vi "Live Capture Functional Stack.6.64bit.vi"() -> ()   [LabVIEW 2014]
uses:
  subvis/Stack Track.ctl
  subvis/Stack_State.ctl
  Desktop/camtiff/ctiff.llb/__CTIFFNewFileAndStyleUINT16.vi
  Desktop/camtiff/ctiff.llb/__CTIFFAddNewPageUINT16.vi
  CameraControlTypeDef.ctl
panel:
  in  "Slit Width / Lines 2":sgl=150.0
  out "Frame Index":i32
  in  "Internal Line Interval":dbl
  in  "Readout Direction":sgl(ring)=1.0 items=["Forward"=1, "Backward"=2]
  in  "Trigger Mode":sgl(ring)=1.0 items=["Normal"=1, "Start "=6]
  in  "Trigger Source":sgl(ring)=2.0 items=["Internal"=1, "External"=2]
  out "State":T1=enum."Start Sequence"
  out "Image":u16[][](graph)
  out "Saving":bool
  in  "AutoIncrement":bool=TRUE
  in  "Path":path=path "C:/Users/spim/Desktop/Craig Cap/temp/a.tiff"
  out "error out":errorcluster
  in  "stop":bool
  out "Total Frames":i32
  out "Elapsed Time":u32
  out "Software FPS":dbl
  out "Camera FPS":dbl
  in  "H Offset":i32 min=0 max=0
  in  "H Width":i32 min=0 max=0
  out "SMD":dbl
  out "SHO":i32
  in  "V Offset":i32 min=0 max=0
  in  "V Width":i32 min=0 max=0
  in  "Binning":u16(ring) items=["1x1"=1, "2x2"=2, "4x4"=4]
  out "SHW":i32
  out "SVO":i32
  out "SVW":i32
  in  "Scan Mode":dbl min=0.0 max=0.0
  in  "Exposure":dbl min=0.0 max=0.0
  out "EXP":dbl
  out "Camera Model":string
  out "Camera Version":string
  out "Camera Serial":string
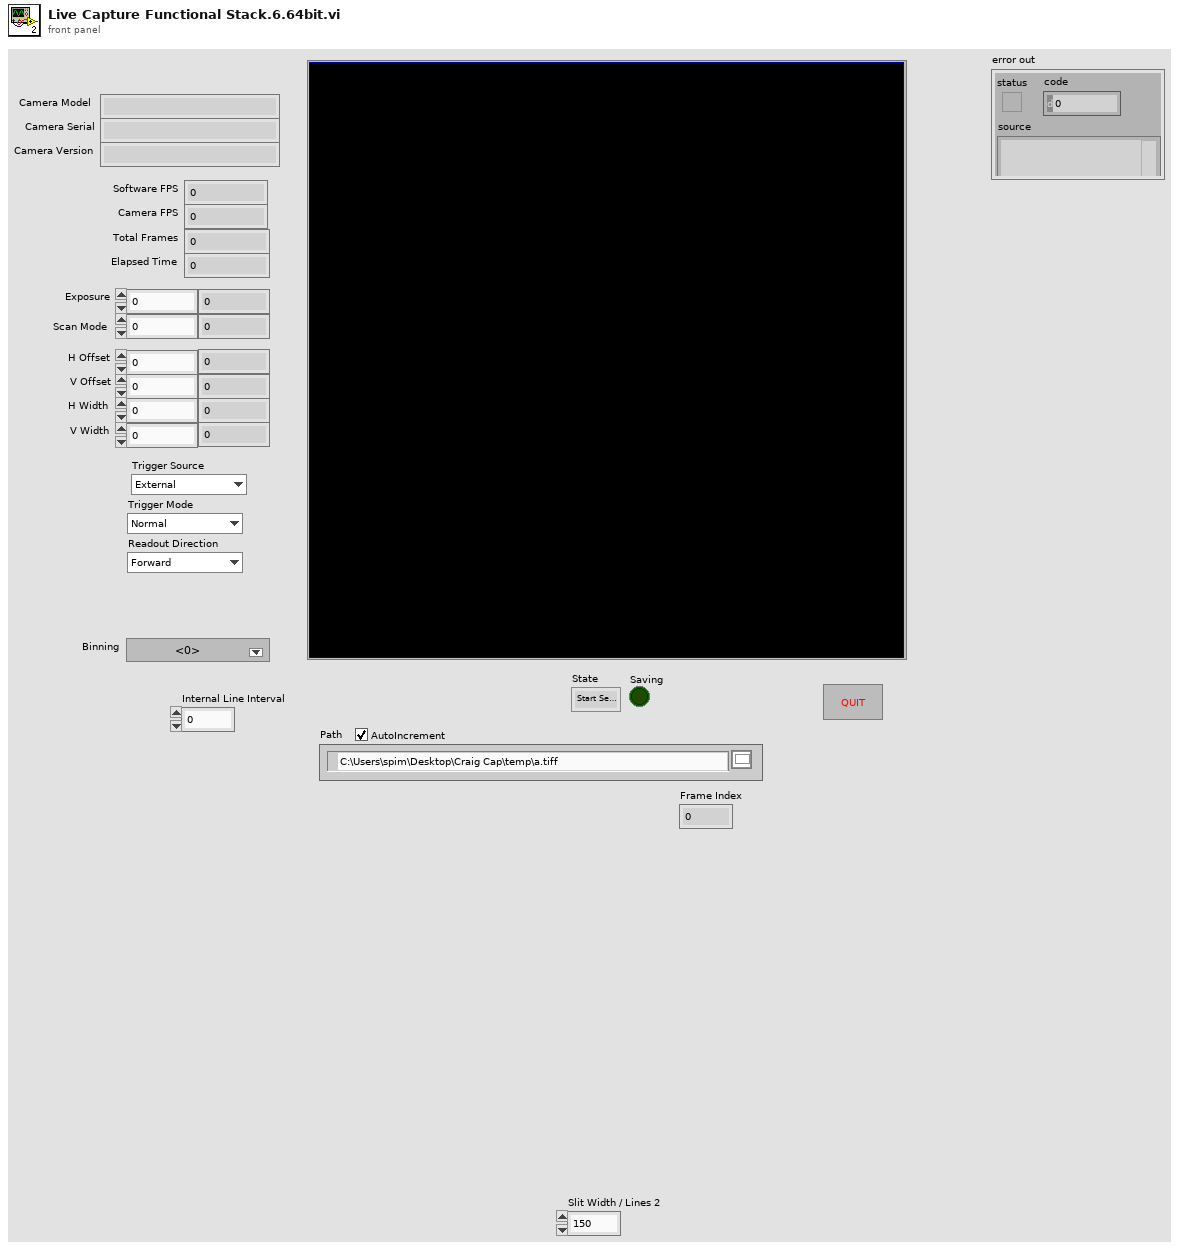
[diagram p1: front panel]
types:
  T1 = typedef "Stack Track.ctl" = enum16{"Idle", "Start Sequence", "Read Disk", "STOP", "Collecting", "End"}
  T2 = typedef "CameraControlTypeDef.ctl" = enum16{"Ram Record", "HardDisk Record", "Disengage Update", "Update", "Idle"}
  T3 = typedef "Stack_State.ctl" = cluster{"State":T1, "Stack Number":i32, "Image":u16[][]}
  T4 = cluster{"Model":string, "Camera ID":string, "Firmware":string}
  T5 = cluster{"Value":i32, "Minimum":i32, "Maximum":i32, "Increment":i32}
  T6 = cluster{"height":u32, "width":u32, "datatype":u32}
  T7 = cluster{"H Offset":i32, "V Offset":i32, "H Width":i32, "V Width":i32}
  T8 = enum8{"Enabled", "Disabled", "Disabled and Grayed Out"}
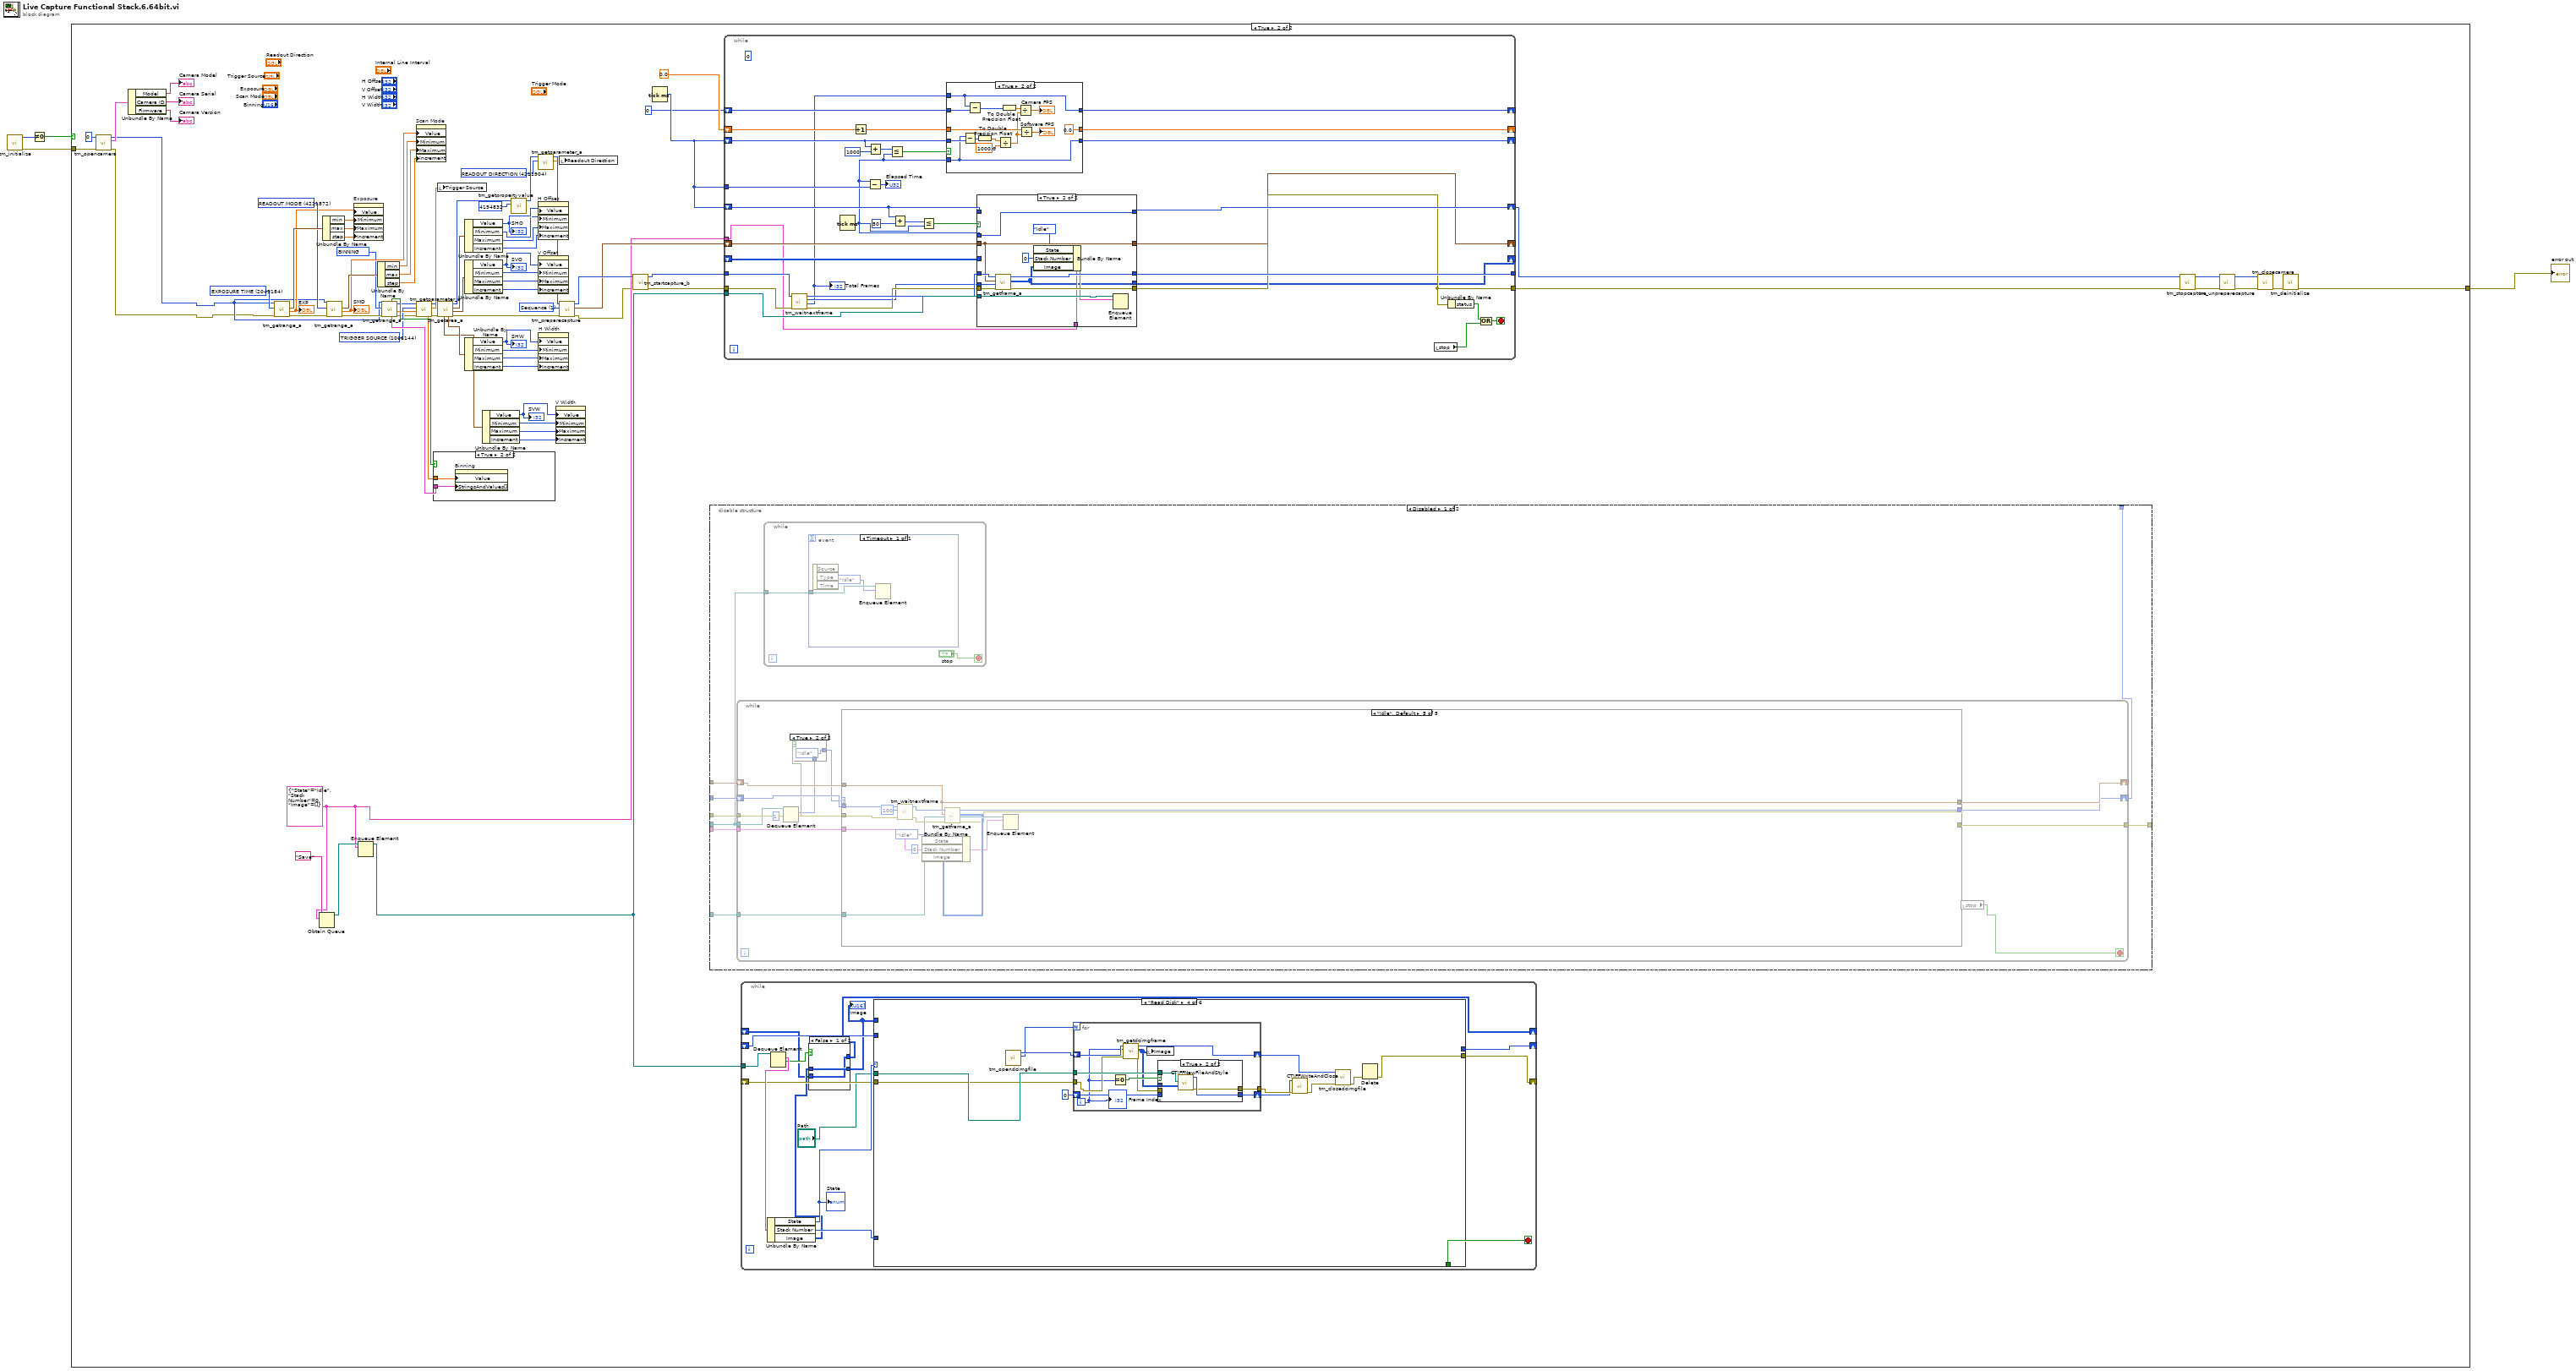
[diagram p0: block diagram]
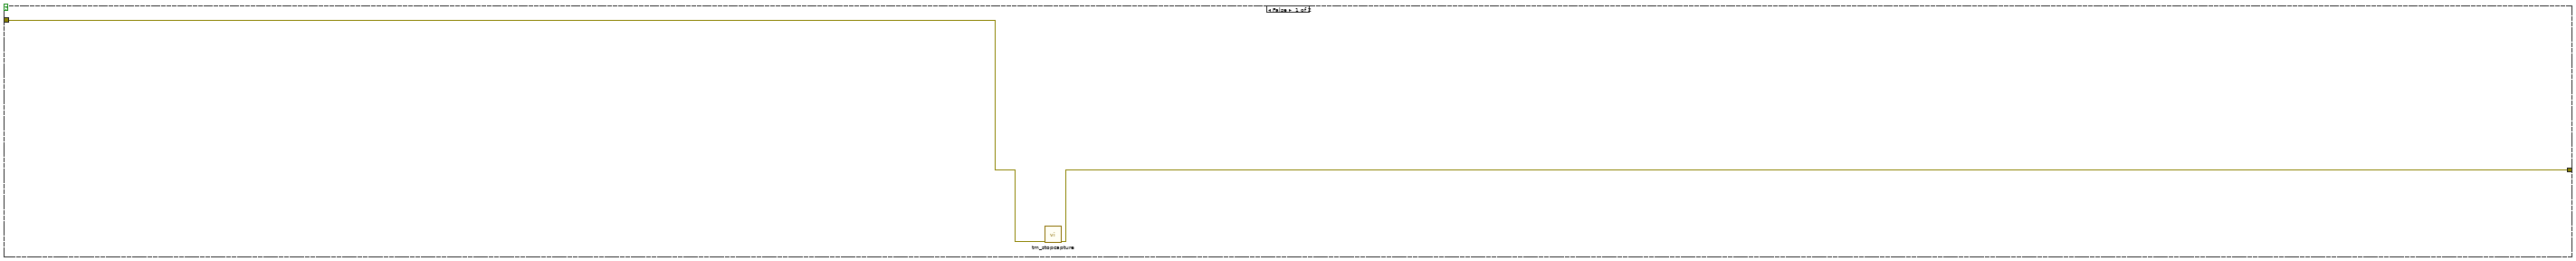
[diagram p2: hidden frame]
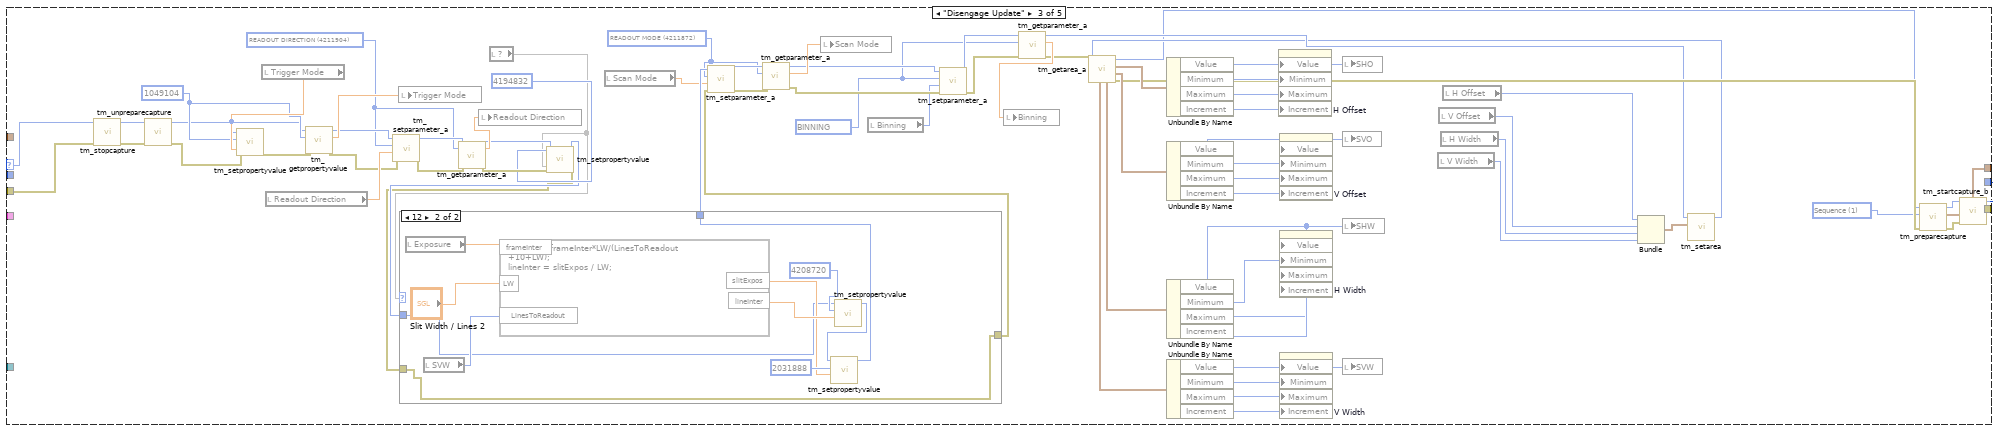
[diagram p8: hidden frame]
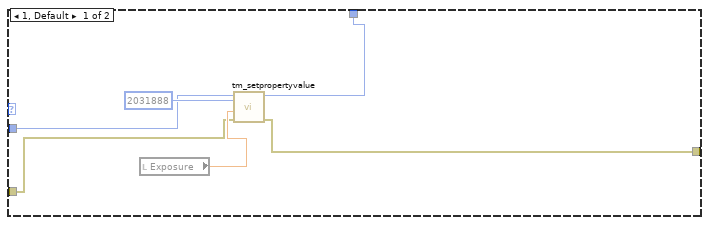
[diagram p9: hidden frame]
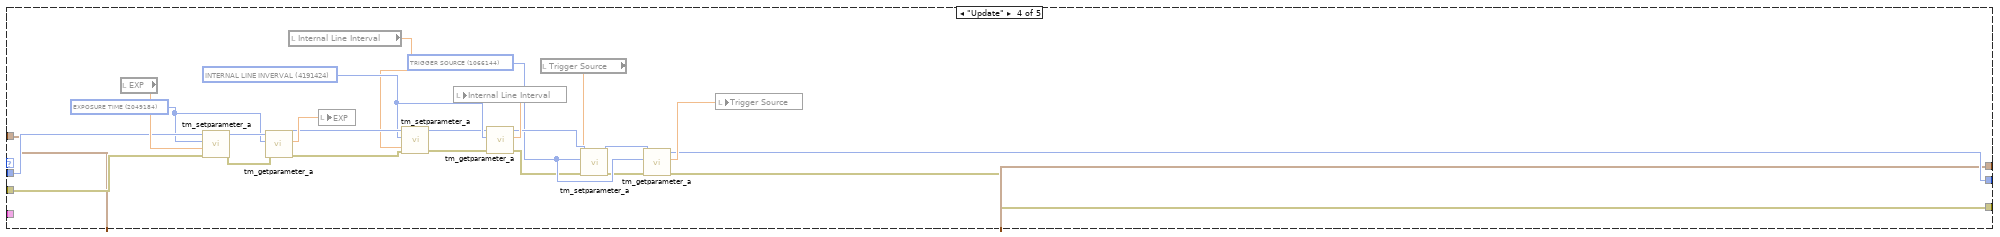
[diagram p10: hidden frame]
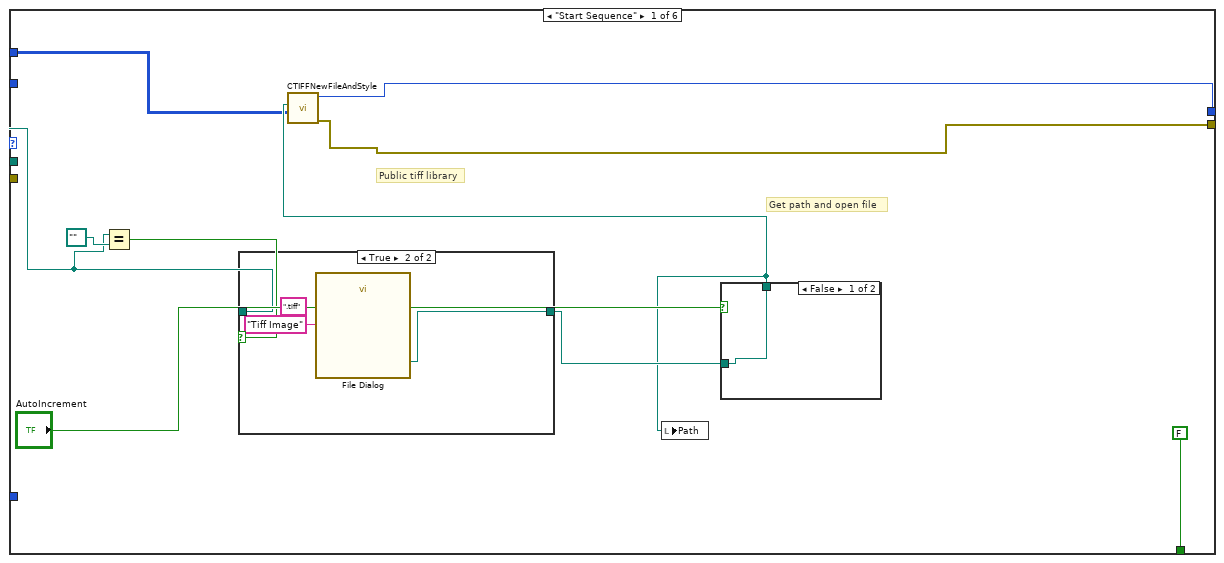
[diagram p13: hidden frame]
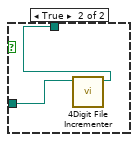
[diagram p15: hidden frame]
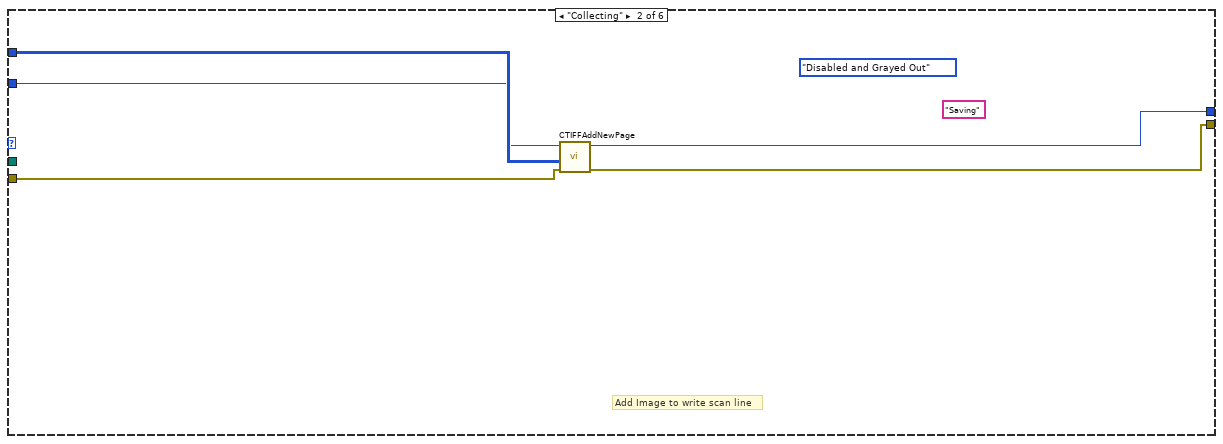
[diagram p16: hidden frame]
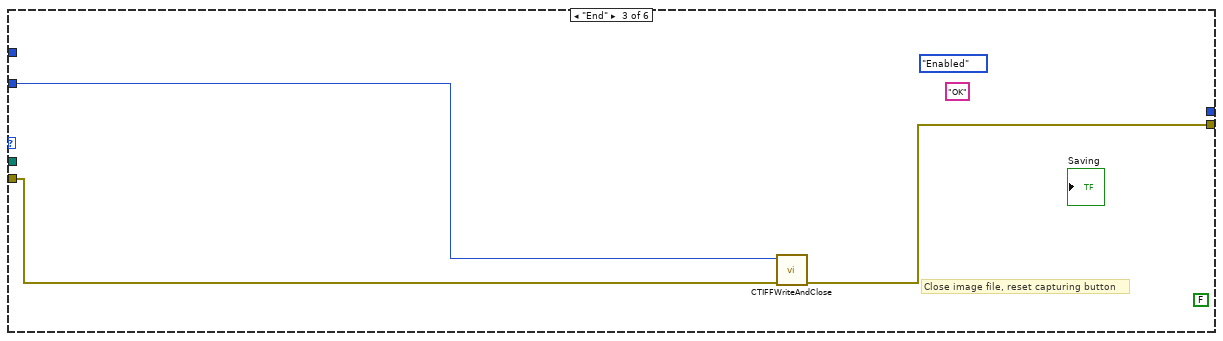
[diagram p17: hidden frame]
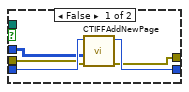
[diagram p18: hidden frame]
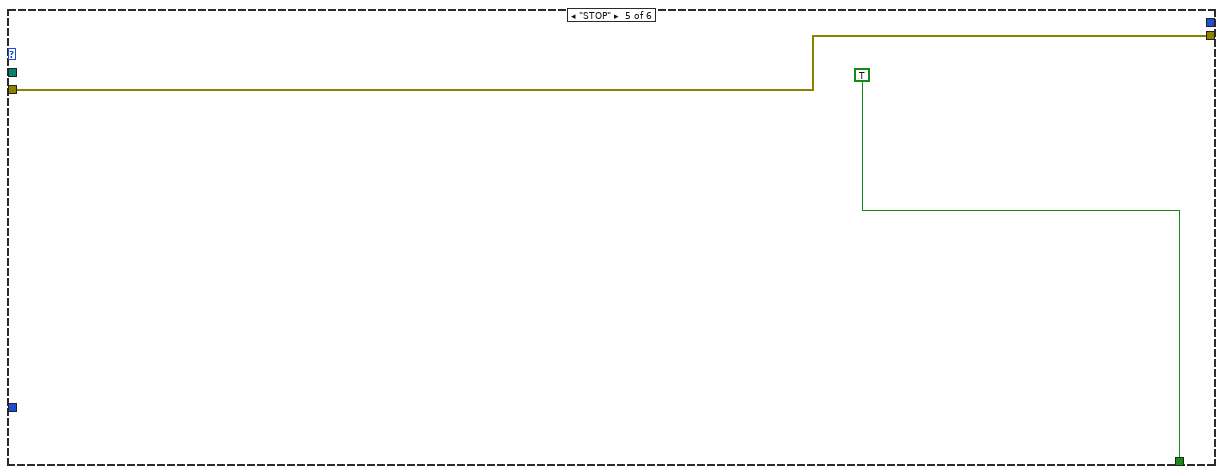
[diagram p19: hidden frame]
diagram:
  n1 = call <userlib>:"tm_initialize.vi"() -> ("error out"=w2:errorcluster, "Number Of Cameras"=w1:u32)  [unwired: 8 in, 2 out]
  n2 = Not Equal To 0?(x=w1) -> (x != 0?=w4:bool)
  n3 = case shown="True" w4 {
    tunnel: [w5 w83] -> w3
    tunnel: w2 -> [w6 w86]
    frame False {
      n4 = call <userlib>:"tm_stopcapture.vi"("error in (no error)"=w6) -> ("error out"=w5:errorcluster)  [unwired: 9 in, 1 out]
    }
    frame True {
      w19 = u32 4211904 items=["SENSOR MODE"=4212128, "CCD MODE"=4212384, "READOUT MODE"=4211872, "ACTIVE VIEW INDEX"=4343136, "BITS PER CHANNEL"=4342976, "IMAGE PIXEL TYPE"=4343296, "BINNING"=4215968, "EXPOSURE TIME"=2049184, "CONTRAST GAIN"=3163312, "CONTRAST OFFSET"=3163328, "LIGHT MODE"=2114720, "SENSITIVITY"=2114992, "PHOTON IMAGING MODE"=2115200, "HIGH DYNAMIC RANGE MODE"=3163360, "WHITE BALANCE"=3163568, "TEMPERATURE"=2115232, "TEMPERATURE TARGET"=2115264, "SENSOR COOLER FAN"=2115296, "LINEBUNDLE HEIGHT"=4212192, "MECHANICAL SHUTTER"=2115488, "BACK FOCUS POSITION"=8422304, "TRIGGER CONNECTOR"=1066432, "TRIGGER SOURCE"=1066144, "OUTPUT TRIGGER SOURCE"=1852576, "TRIGGER GLOBAL EXPOSURE"=2049680, "FIRST TRIGGER BEHAVIOR"=2049696, "CHANNEL SYNC"=1852352, "READOUT DIRECTION"=4211904, "PRE HSYNC COUNT"=1852704] ("Parameter")
      w28 = u32 1066144 items=["SENSOR MODE"=4212128, "CCD MODE"=4212384, "READOUT MODE"=4211872, "ACTIVE VIEW INDEX"=4343136, "BITS PER CHANNEL"=4342976, "IMAGE PIXEL TYPE"=4343296, "BINNING"=4215968, "EXPOSURE TIME"=2049184, "CONTRAST GAIN"=3163312, "CONTRAST OFFSET"=3163328, "LIGHT MODE"=2114720, "SENSITIVITY"=2114992, "PHOTON IMAGING MODE"=2115200, "HIGH DYNAMIC RANGE MODE"=3163360, "WHITE BALANCE"=3163568, "TEMPERATURE"=2115232, "TEMPERATURE TARGET"=2115264, "SENSOR COOLER FAN"=2115296, "LINEBUNDLE HEIGHT"=4212192, "MECHANICAL SHUTTER"=2115488, "BACK FOCUS POSITION"=8422304, "TRIGGER CONNECTOR"=1066432, "TRIGGER SOURCE"=1066144, "OUTPUT TRIGGER SOURCE"=1852576, "TRIGGER GLOBAL EXPOSURE"=2049680, "FIRST TRIGGER BEHAVIOR"=2049696, "CHANNEL SYNC"=1852352, "READOUT DIRECTION"=4211904, "PRE HSYNC COUNT"=1852704] ("Parameter")
      w12 = T3 {"State"=enum."Idle", "Stack Number"=0, "Image"=[]} ("input cluster")
      w33 = u32 2049184 items=["BINNING"=4215968, "BITS PER CHANNEL"=4342976, "ACTIVE VIEW INDEX"=4343136, "CCD MODE"=4212384, "SENSOR MODE"=4212128, "READOUT MODE"=4211872, "EXPOSURE TIME"=2049184, "CONTRAST GAIN"=3163312, "CONTRAST OFFSET"=3163328, "LIGHT MODE"=2114720, "SENSITIVITY"=2114992, "WHITE BALANCE"=3163568, "PHOTON IMAGING MODE"=2115200, "HIGH DYNAMIC RANGE MODE"=3163360, "TRIGGER SOURCE"=1066144, "TRIGGER ACTIVE"=1066160, "TRIGGER MODE"=1066400, "TRIGGER POLARITY"=1066416, "TRIGGER GLOBAL EXPOSURE"=2049680, "FIRST TRIGGER BEHAVIOR"=2049696, "TRIGGER TIMES"=1066448, "OUTPUT TRIGGER POLARITY"=1852592, "OUTPUT TRIGGER DELAY"=1852624, "OUTPUT TRIGGER PERIOD"=1852640, "TEMPERATURE"=2115232, "TEMPERATURE TARGET"=2115264, "SENSOR COOLER FAN"=2115296, "MECHANICAL SHUTTER"=2115488, "BACK FOCUS POSITION"=8422304, "FRAMEBUNDLE MODE"=4346784, "FRAMEBUNDLE NUMBER"=4346800, "LINEBUNDLE HEIGHT"=4212192, "TRIGGER CONNECTOR"=1066432, "IMAGE PIXEL TYPE"=4343296, "OUTPUT TRIGGER KIND"=1852656, "READOUT DIRECTION"=4211904, "CHANNEL SYNC"=1852352] ("Parameter")
      w34 = u32 4211872 items=["BINNING"=4215968, "BITS PER CHANNEL"=4342976, "ACTIVE VIEW INDEX"=4343136, "CCD MODE"=4212384, "SENSOR MODE"=4212128, "READOUT MODE"=4211872, "EXPOSURE TIME"=2049184, "CONTRAST GAIN"=3163312, "CONTRAST OFFSET"=3163328, "LIGHT MODE"=2114720, "SENSITIVITY"=2114992, "WHITE BALANCE"=3163568, "PHOTON IMAGING MODE"=2115200, "HIGH DYNAMIC RANGE MODE"=3163360, "TRIGGER SOURCE"=1066144, "TRIGGER ACTIVE"=1066160, "TRIGGER MODE"=1066400, "TRIGGER POLARITY"=1066416, "TRIGGER GLOBAL EXPOSURE"=2049680, "FIRST TRIGGER BEHAVIOR"=2049696, "TRIGGER TIMES"=1066448, "OUTPUT TRIGGER POLARITY"=1852592, "OUTPUT TRIGGER DELAY"=1852624, "OUTPUT TRIGGER PERIOD"=1852640, "TEMPERATURE"=2115232, "TEMPERATURE TARGET"=2115264, "SENSOR COOLER FAN"=2115296, "MECHANICAL SHUTTER"=2115488, "BACK FOCUS POSITION"=8422304, "FRAMEBUNDLE MODE"=4346784, "FRAMEBUNDLE NUMBER"=4346800, "LINEBUNDLE HEIGHT"=4212192, "TRIGGER CONNECTOR"=1066432, "IMAGE PIXEL TYPE"=4343296, "OUTPUT TRIGGER KIND"=1852656, "READOUT DIRECTION"=4211904, "CHANNEL SYNC"=1852352] ("Parameter")
      w35 = u32 4215968 items=["BINNING"=4215968, "BITS PER CHANNEL"=4342976, "ACTIVE VIEW INDEX"=4343136, "CCD MODE"=4212384, "SENSOR MODE"=4212128, "READOUT MODE"=4211872, "EXPOSURE TIME"=2049184, "CONTRAST GAIN"=3163312, "CONTRAST OFFSET"=3163328, "LIGHT MODE"=2114720, "SENSITIVITY"=2114992, "WHITE BALANCE"=3163568, "PHOTON IMAGING MODE"=2115200, "HIGH DYNAMIC RANGE MODE"=3163360, "TRIGGER SOURCE"=1066144, "TRIGGER ACTIVE"=1066160, "TRIGGER MODE"=1066400, "TRIGGER POLARITY"=1066416, "TRIGGER GLOBAL EXPOSURE"=2049680, "FIRST TRIGGER BEHAVIOR"=2049696, "TRIGGER TIMES"=1066448, "OUTPUT TRIGGER POLARITY"=1852592, "OUTPUT TRIGGER DELAY"=1852624, "OUTPUT TRIGGER PERIOD"=1852640, "TEMPERATURE"=2115232, "TEMPERATURE TARGET"=2115264, "SENSOR COOLER FAN"=2115296, "MECHANICAL SHUTTER"=2115488, "BACK FOCUS POSITION"=8422304, "FRAMEBUNDLE MODE"=4346784, "FRAMEBUNDLE NUMBER"=4346800, "LINEBUNDLE HEIGHT"=4212192, "TRIGGER CONNECTOR"=1066432, "IMAGE PIXEL TYPE"=4343296, "OUTPUT TRIGGER KIND"=1852656, "READOUT DIRECTION"=4211904, "CHANNEL SYNC"=1852352] ("Parameter")
      w81 = 1 items=["Snap", "Sequence"] ("Capture mode")
      n5 = call <userlib>:"tm_opencamera.vi"("error in (no error)"=w86, "Camera Index"=u32 0) -> ("error out"=w7:errorcluster, "Camera Details"=w47:T4, "Handle out"=w8:u32)  [unwired: 7 in]
      n6 = Unbundle By Name(w47) -> ("Model"=→"Camera Model":string, "Camera ID"=→"Camera Serial":string, "Firmware"=→"Camera Version":string)
      n7 = call <userlib>:"tm_getrange_a.vi"("error in (no error)"=w7, "Parameter"=w33, "Handle in"=w8) -> ("error out"=w42:errorcluster, "default"=w31:dbl, "Range"=w43:cluster{"min":dbl, "max":dbl, "step":dbl})  [unwired: 2 in, 4 out]
      "EXP" <- w31
      n8 = Obtain Queue(name (unnamed)="Save", element data type=w12) -> (queue out=w16:refnum<queue>)  [unwired: 3 in, 2 out]
      n9 = Unbundle By Name(w43) -> ("min"=w78:dbl, "max"=w77:dbl, "step"=w76:dbl)
      n10 = call <userlib>:"tm_getrange_a.vi"("error in (no error)"=w42, "Parameter"=w34, "Handle in"=w8) -> ("error out"=w39:errorcluster, "default"=w40:dbl, "Range"=w41:cluster{"min":dbl, "max":dbl, "step":dbl})  [unwired: 2 in, 4 out]
      "SMD" <- w40
      n11 = property on="Exposure" class="DigNum (strict)"("Value"=w31, "Minimum"=w78, "Maximum"=w77, "Increment"=w76) -> ()  [unwired: 2 in, 2 out]
      n12 = Enqueue Element(queue=w16, element=w12) -> (queue out=w15:refnum<queue>)  [unwired: 2 in, 2 out]
      n13 = Unbundle By Name(w41) -> ("min"=w75:dbl, "max"=w74:dbl, "step"=w73:dbl)
      n14 = call <userlib>:"tm_getrange_a.vi"("error in (no error)"=w39, "Parameter"=w35, "Handle in"=w8) -> ("error out"=w25:errorcluster, "default"=w37:dbl, "Handle out"=w27:u32, "Value Names"=w36:cluster{"Name":string, "Value":dbl}[], "Writable"=w38:bool)  [unwired: 2 in, 2 out]
      n15 = property on="Scan Mode" class="DigNum (strict)"("Value"=w40, "Minimum"=w75, "Maximum"=w74, "Increment"=w73) -> ()  [unwired: 2 in, 2 out]
      n16 = call <userlib>:"tm_getparameter_a.vi"("error in (no error)"=w25, "Parameter"=w28, "Handle in"=w27) -> ("error out"=w24:errorcluster, "Value out"=w29:dbl, "Handle out"=w26:u32)  [unwired: 6 in]
      n17 = case shown="True" w38 {
        tunnel: w36 -> [_ w398]
        tunnel: w37 -> [_ w397]
        frame False {
        }
        frame True {
          n18 = property on="Binning" class="Ring (strict)"("Value"=w397, "StringsAndValues[]"=w398) -> ()  [unwired: 2 in, 2 out]
        }
      }
      n19 = local write "Trigger Source"(w29) -> ()
      n20 = call <userlib>:"tm_getarea_a.vi"("error in (no error)"=w24, "Handle in"=w26) -> ("error out"=w30:errorcluster, "V Offset"=w72:T5, "H Offset"=w53:T5, "Handle out"=w22:u32, "H Width"=w71:T5, "V Width"=w70:T5)  [unwired: 4 in]
      n21 = Unbundle By Name(w53) -> ("Value"=w52:i32, "Minimum"=w51:i32, "Maximum"=w50:i32, "Increment"=w49:i32)
      "SHO" <- w52
      n22 = Unbundle By Name(w72) -> ("Value"=w60:i32, "Minimum"=w69:i32, "Maximum"=w68:i32, "Increment"=w67:i32)
      "SVO" <- w60
      n23 = Unbundle By Name(w71) -> ("Value"=w59:i32, "Minimum"=w66:i32, "Maximum"=w65:i32, "Increment"=w64:i32)
      "SHW" <- w59
      n24 = Unbundle By Name(w70) -> ("Value"=w58:i32, "Minimum"=w63:i32, "Maximum"=w62:i32, "Increment"=w61:i32)
      "SVW" <- w58
      n25 = call <userlib>:"tm_getpropertyvalue.vi"("Property ID"=u32 4194832, "Handle in"=w22) -> ("Handle out"=w21:u32)  [unwired: 7 in, 2 out]
      n26 = call <userlib>:"tm_getparameter_a.vi"("Parameter"=w19, "Handle in"=w21) -> ("Value out"=w18:dbl, "Handle out"=w20:u32)  [unwired: 7 in, 1 out]
      n27 = property on="H Offset" class="DigNum (strict)"("Value"=w52, "Minimum"=w51, "Maximum"=w50, "Increment"=w49) -> ()  [unwired: 2 in, 2 out]
      n28 = property on="V Offset" class="DigNum (strict)"("Value"=w60, "Minimum"=w69, "Maximum"=w68, "Increment"=w67) -> ()  [unwired: 2 in, 2 out]
      n29 = property on="H Width" class="DigNum (strict)"("Value"=w59, "Minimum"=w66, "Maximum"=w65, "Increment"=w64) -> ()  [unwired: 2 in, 2 out]
      n30 = property on="V Width" class="DigNum (strict)"("Value"=w58, "Minimum"=w63, "Maximum"=w62, "Increment"=w61) -> ()  [unwired: 2 in, 2 out]
      n31 = local write "Readout Direction"(w18) -> ()
      n32 = call <userlib>:"tm_preparecapture.vi"("error in (no error)"=w30, "Capture mode"=w81, "Handle in"=w20) -> ("error out"=w11:errorcluster, "Buffer Info"=w13:T6, "Handle out"=w17:u32)  [unwired: 5 in, 1 out]
      n33 = call <userlib>:"tm_startcapture_b.vi"("error in (no error)"=w11, "Handle in"=w17) -> ("error out"=w80:errorcluster, "Handle out"=w14:u32)  [unwired: 8 in]
      n34 = Tick Count (ms)() -> (millisecond timer value=w79:u32)
      n35 = disable-structure shown="Disabled" {
        disable-tunnel: _ -> [w164 _]
        disable-tunnel: _ -> [w163 _]
        disable-tunnel: _ -> [w162 _]
        disable-tunnel: _ -> [w161 _]
        disable-tunnel: _ -> [w160 _]
        disable-tunnel: [w159 _] -> _
        disable-tunnel: [w158 _] -> _
        disable-tunnel: _ -> [w157 _]
        frame Disabled {
          n36 = while {
            tunnel: w164 -> [w179]
            tunnel: w157 -> [w182]
            tunnel: w161 -> [w178]
            shift-right: [w177] -> _
            shift-left: w162 -> [w180]
            shift-right: [w176] -> w158
            shift-left: w163 -> [w181]
            tunnel: w160 -> [w175]
            tunnel: [w174] -> w159
            stop <- w169 stop-if-true
            n37 = Dequeue Element(queue=w182, timeout in ms (-1)=1) -> (element=w170:T2, timed out?=w172:bool)  [unwired: 1 in, 2 out]
            n38 = case shown="True" w172 {
              tunnel: [w183 CameraControlTypeDef."Idle" ("Enum")] -> w171
              tunnel: w170 -> [w183 _]
              frame False {
              }
              frame True {
              }
            }
            n39 = case shown="\"Idle\", Default" w171 {
              selector: w171 -> [_ _ w263 _ _]
              tunnel: w181 -> [w187 w188 _ w301 w318]
              tunnel: w180 -> [w186 w190 _ w286 w310]
              tunnel: w179 -> [_ _ _ _ w316]
              tunnel: w178 -> [_ _ _ _ w315]
              tunnel: [w186 w190 w201 w286 w310] -> w177
              tunnel: [w187 w188 w191 w287 w309] -> w176
              tunnel: w175 -> [w185 w189 w260 w300 w306]
              tunnel: [w185 w189 w200 w285 w308] -> w174
              frame "Ram Record" {
              }
              frame "HardDisk Record" {
              }
              frame "Disengage Update" {
                w204 = 1 items=["Snap", "Sequence"] ("Capture mode")
                w207 = u32 4215968 items=["BINNING"=4215968, "BITS PER CHANNEL"=2, "ACTIVE VIEW INDEX"=3, "CCD MODE"=4, "SENSOR MODE"=5, "READOUT MODE"=6, "EXPOSURE TIME"=7, "CONTRAST GAIN"=8, "CONTRAST OFFSET"=9, "LIGHT MODE"=10, "SENSITIVITY"=11, "WHITE BALANCE"=12, "PHOTON IMAGING MODE"=13, "HIGH DYNAMIC RANGE MODE"=14, "TRIGGER SOURCE"=15, "TRIGGER ACTIVE"=16, "TRIGGER MODE"=17, "TRIGGER POLARITY"=18, "TRIGGER GLOBAL EXPOSURE"=19, "FIRST TRIGGER BEHAVIOR"=20, "TRIGGER TIMES"=21, "OUTPUT TRIGGER POLARITY"=22, "OUTPUT TRIGGER DELAY"=23, "OUTPUT TRIGGER PERIOD"=24, "TEMPERATURE"=25, "TEMPERATURE TARGET"=26, "SENSOR COOLER FAN"=27, "MECHANICAL SHUTTER"=28, "BACK FOCUS POSITION"=29, "FRAMEBUNDLE MODE"=30, "FRAMEBUNDLE NUMBER"=31, "LINEBUNDLE HEIGHT"=32, "TRIGGER CONNECTOR"=33, "IMAGE PIXEL TYPE"=34, "OUTPUT TRIGGER KIND"=35, "READOUT DIRECTION"=36, "CHANNEL SYNC"=37] ("Parameter")
                w234 = u32 4211872 items=["SENSOR MODE"=4212128, "CCD MODE"=4212384, "READOUT MODE"=4211872, "ACTIVE VIEW INDEX"=4343136, "BITS PER CHANNEL"=4342976, "IMAGE PIXEL TYPE"=4343296, "BINNING"=4215968, "EXPOSURE TIME"=2049184, "CONTRAST GAIN"=3163312, "CONTRAST OFFSET"=3163328, "LIGHT MODE"=2114720, "SENSITIVITY"=2114992, "PHOTON IMAGING MODE"=2115200, "HIGH DYNAMIC RANGE MODE"=3163360, "WHITE BALANCE"=3163568, "TEMPERATURE"=2115232, "TEMPERATURE TARGET"=2115264, "SENSOR COOLER FAN"=2115296, "LINEBUNDLE HEIGHT"=4212192, "MECHANICAL SHUTTER"=2115488, "BACK FOCUS POSITION"=8422304, "TRIGGER CONNECTOR"=1066432, "TRIGGER SOURCE"=1066144, "OUTPUT TRIGGER SOURCE"=1852576, "TRIGGER GLOBAL EXPOSURE"=2049680, "FIRST TRIGGER BEHAVIOR"=2049696, "CHANNEL SYNC"=1852352, "READOUT DIRECTION"=4211904, "PRE HSYNC COUNT"=1852704] ("Parameter")
                w247 = u32 4211904 items=["SENSOR MODE"=4212128, "CCD MODE"=4212384, "READOUT MODE"=4211872, "ACTIVE VIEW INDEX"=4343136, "BITS PER CHANNEL"=4342976, "IMAGE PIXEL TYPE"=4343296, "BINNING"=4215968, "EXPOSURE TIME"=2049184, "CONTRAST GAIN"=3163312, "CONTRAST OFFSET"=3163328, "LIGHT MODE"=2114720, "SENSITIVITY"=2114992, "PHOTON IMAGING MODE"=2115200, "HIGH DYNAMIC RANGE MODE"=3163360, "WHITE BALANCE"=3163568, "TEMPERATURE"=2115232, "TEMPERATURE TARGET"=2115264, "SENSOR COOLER FAN"=2115296, "LINEBUNDLE HEIGHT"=4212192, "MECHANICAL SHUTTER"=2115488, "BACK FOCUS POSITION"=8422304, "TRIGGER CONNECTOR"=1066432, "TRIGGER SOURCE"=1066144, "OUTPUT TRIGGER SOURCE"=1852576, "TRIGGER GLOBAL EXPOSURE"=2049680, "FIRST TRIGGER BEHAVIOR"=2049696, "CHANNEL SYNC"=1852352, "READOUT DIRECTION"=4211904, "PRE HSYNC COUNT"=1852704] ("Parameter")
                w258 = u32 1049104 ("Property ID")
                n40 = call <userlib>:"tm_stopcapture.vi"("error in (no error)"=w260, "Handle in"=w263) -> ("error out"=w261:errorcluster, "Handle out"=w262:u32)  [unwired: 8 in]
                n41 = call <userlib>:"tm_unpreparecapture.vi"("error in (no error)"=w261, "Handle in"=w262) -> ("error out"=w249:errorcluster, "Handle out"=w257:u32)  [unwired: 8 in]
                n42 = local read "Trigger Mode"() -> (w259:sgl)
                n43 = call <userlib>:"tm_setpropertyvalue.vi"("error in (no error)"=w249, "Value in"=w259, "Property ID"=w258, "Handle in"=w257) -> ("error out"=w250:errorcluster)  [unwired: 6 in, 1 out]
                n44 = local read "Readout Direction"() -> (w254:sgl)
                n45 = call <userlib>:"tm_getpropertyvalue.vi"("error in (no error)"=w250, "Property ID"=w258, "Handle in"=w257) -> ("error out"=w251:errorcluster, "Value in"=w256:sgl, "Handle out"=w255:u32)  [unwired: 6 in]
                n46 = call <userlib>:"tm_setparameter_a.vi"("error in (no error)"=w251, "Value in"=w254, "Parameter"=w247, "Handle in"=w255) -> ("error out"=w252:errorcluster, "Handle out"=w253:u32)  [unwired: 6 in]
                n47 = local write "Trigger Mode"(w256) -> ()
                n48 = call <userlib>:"tm_getparameter_a.vi"("error in (no error)"=w252, "Parameter"=w247, "Handle in"=w253) -> ("error out"=w245:errorcluster, "Value out"=w248:dbl, "Handle out"=w246:u32)  [unwired: 6 in]
                n49 = local write "Readout Direction"(w248) -> ()
                n50 = local read item#-1() -> (w243)
                n51 = call <userlib>:"tm_setpropertyvalue.vi"("error in (no error)"=w245, "Value in"=w243, "Property ID"=u32 4194832, "Handle in"=w246) -> ("error out"=w241:errorcluster, "Handle out"=w242:u32)  [unwired: 6 in]
                n52 = case shown="12" w243 {
                  tunnel: [w267 w271] -> w240
                  tunnel: w242 -> [w266 w272]
                  tunnel: w241 -> [w265 w271]
                  tunnel: [w264 w270] -> w238
                  frame 1, Default {
                    n53 = local read "Exposure"() -> (w268:dbl)
                    n54 = call <userlib>:"tm_setpropertyvalue.vi"("error in (no error)"=w265, "Value in"=w268, "Property ID"=u32 2031888, "Handle in"=w266) -> ("error out"=w267:errorcluster, "Handle out"=w264:u32)  [unwired: 6 in]
                  }
                  frame 12 {
                    n55 = local read "Exposure"() -> (w280:dbl)
                    n56 = local read "SVW"() -> (w278:i32)
                    n57 = formula code="slitExpos=frameInter*LW/(LinesToReadout\n+10+LW);\nlineInter = slitExpos / LW;"("frameInter"=w280, "LW"="Slit Width / Lines 2", "LinesToReadout"=w278) -> ("slitExpos"=w273:dbl, "lineInter"=w276:dbl)
                    n58 = call <userlib>:"tm_setpropertyvalue.vi"("Value in"=w276, "Property ID"=u32 4208720, "Handle in"=w272) -> ("Handle out"=w275:u32)  [unwired: 7 in, 1 out]
                    n59 = call <userlib>:"tm_setpropertyvalue.vi"("Value in"=w273, "Property ID"=u32 2031888, "Handle in"=w275) -> ("Handle out"=w270:u32)  [unwired: 7 in, 1 out]
                  }
                }
                n60 = local read "Scan Mode"() -> (w237:dbl)
                n61 = call <userlib>:"tm_setparameter_a.vi"("error in (no error)"=w240, "Value in"=w237, "Parameter"=w234, "Handle in"=w238) -> ("error out"=w239:errorcluster, "Handle out"=w235:u32)  [unwired: 6 in]
                n62 = call <userlib>:"tm_getparameter_a.vi"("error in (no error)"=w239, "Parameter"=w234, "Handle in"=w235) -> ("error out"=w233:errorcluster, "Value out"=w236:dbl, "Handle out"=w232:u32)  [unwired: 6 in]
                n63 = local write "Scan Mode"(w236) -> ()
                n64 = local read "Binning"() -> (w231:u16)
                n65 = call <userlib>:"tm_setparameter_a.vi"("error in (no error)"=w233, "Value in"=w231, "Parameter"=w207, "Handle in"=w232) -> ("error out"=w210:errorcluster, "Handle out"=w209:u32)  [unwired: 6 in]
                n66 = call <userlib>:"tm_getparameter_a.vi"("error in (no error)"=w210, "Parameter"=w207, "Handle in"=w209) -> ("error out"=w206:errorcluster, "Value out"=w208:dbl, "Handle out"=w194:u32)  [unwired: 6 in]
                n67 = local write "Binning"(w208) -> ()
                n68 = local read "V Width"() -> (w196:i32)
                n69 = local read "V Offset"() -> (w198:i32)
                n70 = local read "H Width"() -> (w197:i32)
                n71 = local read "H Offset"() -> (w199:i32)
                n72 = Bundle("H Offset"=w199, "V Offset"=w198, "H Width"=w197, "V Width"=w196) -> (w195:T7)  [unwired: 1 in]
                n73 = call <userlib>:"tm_setarea.vi"("Sub Region"=w195, "Handle in"=w194) -> ("Handle out"=w193:u32)  [unwired: 8 in, 1 out]
                n74 = call <userlib>:"tm_getarea_a.vi"("error in (no error)"=w206, "Handle in"=w193) -> ("error out"=w205:errorcluster, "V Offset"=w213:T5, "H Offset"=w214:T5, "Handle out"=w192:u32, "H Width"=w212:T5, "V Width"=w211:T5)  [unwired: 4 in]
                n75 = Unbundle By Name(w214) -> ("Value"=w218:i32, "Minimum"=w215:i32, "Maximum"=w216:i32, "Increment"=w217:i32)
                n76 = Unbundle By Name(w213) -> ("Value"=w228:i32, "Minimum"=w219:i32, "Maximum"=w220:i32, "Increment"=w221:i32)
                n77 = Unbundle By Name(w212) -> ("Value"=w229:i32, "Minimum"=w222:i32, "Maximum"=w223:i32, "Increment"=w224:i32)
                n78 = Unbundle By Name(w211) -> ("Value"=w230:i32, "Minimum"=w225:i32, "Maximum"=w226:i32, "Increment"=w227:i32)
                n79 = property on="H Offset" class="DigNum (strict)"("Value"=w218, "Minimum"=w215, "Maximum"=w216, "Increment"=w217) -> ()  [unwired: 2 in, 2 out]
                n80 = property on="V Offset" class="DigNum (strict)"("Value"=w228, "Minimum"=w219, "Maximum"=w220, "Increment"=w221) -> ()  [unwired: 2 in, 2 out]
                n81 = property on="H Width" class="DigNum (strict)"("Value"=w229, "Minimum"=w222, "Maximum"=w223, "Increment"=w224) -> ()  [unwired: 2 in, 2 out]
                n82 = property on="V Width" class="DigNum (strict)"("Value"=w230, "Minimum"=w225, "Maximum"=w226, "Increment"=w227) -> ()  [unwired: 2 in, 2 out]
                n83 = local write "SHO"(w218) -> ()
                n84 = local write "SVO"(w228) -> ()
                n85 = local write "SHW"(w229) -> ()
                n86 = local write "SVW"(w230) -> ()
                n87 = call <userlib>:"tm_preparecapture.vi"("error in (no error)"=w205, "Capture mode"=w204, "Handle in"=w192) -> ("error out"=w203:errorcluster, "Buffer Info"=w201:T6, "Handle out"=w202:u32)  [unwired: 5 in, 1 out]
                n88 = call <userlib>:"tm_startcapture_b.vi"("error in (no error)"=w203, "Handle in"=w202) -> ("error out"=w200:errorcluster, "Handle out"=w191:u32)  [unwired: 8 in]
              }
              frame "Update" {
                w291 = u32 1066144 items=["SENSOR MODE"=4212128, "CCD MODE"=4212384, "READOUT MODE"=4211872, "ACTIVE VIEW INDEX"=4343136, "BITS PER CHANNEL"=4342976, "IMAGE PIXEL TYPE"=4343296, "BINNING"=4215968, "EXPOSURE TIME"=2049184, "CONTRAST GAIN"=3163312, "CONTRAST OFFSET"=3163328, "LIGHT MODE"=2114720, "SENSITIVITY"=2114992, "PHOTON IMAGING MODE"=2115200, "HIGH DYNAMIC RANGE MODE"=3163360, "WHITE BALANCE"=3163568, "TEMPERATURE"=2115232, "TEMPERATURE TARGET"=2115264, "SENSOR COOLER FAN"=2115296, "LINEBUNDLE HEIGHT"=4212192, "MECHANICAL SHUTTER"=2115488, "BACK FOCUS POSITION"=8422304, "TRIGGER CONNECTOR"=1066432, "TRIGGER SOURCE"=1066144, "OUTPUT TRIGGER SOURCE"=1852576, "TRIGGER GLOBAL EXPOSURE"=2049680, "FIRST TRIGGER BEHAVIOR"=2049696, "CHANNEL SYNC"=1852352, "READOUT DIRECTION"=4211904, "PRE HSYNC COUNT"=1852704] ("Parameter")
                w296 = u32 4191424 items=["SENSOR MODE"=4212128, "CCD MODE"=4212384, "READOUT MODE"=4211872, "ACTIVE VIEW INDEX"=4343136, "BITS PER CHANNEL"=4342976, "IMAGE PIXEL TYPE"=4343296, "BINNING"=4215968, "EXPOSURE TIME"=2049184, "CONTRAST GAIN"=3163312, "CONTRAST OFFSET"=3163328, "LIGHT MODE"=2114720, "SENSITIVITY"=2114992, "PHOTON IMAGING MODE"=2115200, "HIGH DYNAMIC RANGE MODE"=3163360, "WHITE BALANCE"=3163568, "TEMPERATURE"=2115232, "TEMPERATURE TARGET"=2115264, "SENSOR COOLER FAN"=2115296, "LINEBUNDLE HEIGHT"=4212192, "MECHANICAL SHUTTER"=2115488, "BACK FOCUS POSITION"=8422304, "TRIGGER CONNECTOR"=1066432, "TRIGGER SOURCE"=1066144, "OUTPUT TRIGGER SOURCE"=1852576, "TRIGGER GLOBAL EXPOSURE"=2049680, "FIRST TRIGGER BEHAVIOR"=2049696, "CHANNEL SYNC"=1852352, "READOUT DIRECTION"=4211904, "PRE HSYNC COUNT"=1852704, "INTERNAL LINE SPEED"=4191408, "INTERNAL LINE INVERVAL"=4191424] ("Parameter")
                w297 = u32 2049184 items=["SENSOR MODE"=4212128, "CCD MODE"=4212384, "READOUT MODE"=4211872, "ACTIVE VIEW INDEX"=4343136, "BITS PER CHANNEL"=4342976, "IMAGE PIXEL TYPE"=4343296, "BINNING"=4215968, "EXPOSURE TIME"=2049184, "CONTRAST GAIN"=3163312, "CONTRAST OFFSET"=3163328, "LIGHT MODE"=2114720, "SENSITIVITY"=2114992, "PHOTON IMAGING MODE"=2115200, "HIGH DYNAMIC RANGE MODE"=3163360, "WHITE BALANCE"=3163568, "TEMPERATURE"=2115232, "TEMPERATURE TARGET"=2115264, "SENSOR COOLER FAN"=2115296, "LINEBUNDLE HEIGHT"=4212192, "MECHANICAL SHUTTER"=2115488, "BACK FOCUS POSITION"=8422304, "TRIGGER CONNECTOR"=1066432, "TRIGGER SOURCE"=1066144, "OUTPUT TRIGGER SOURCE"=1852576, "TRIGGER GLOBAL EXPOSURE"=2049680, "FIRST TRIGGER BEHAVIOR"=2049696, "CHANNEL SYNC"=1852352, "READOUT DIRECTION"=4211904, "PRE HSYNC COUNT"=1852704] ("Parameter")
                n89 = local read "EXP"() -> (w302:dbl)
                n90 = call <userlib>:"tm_setparameter_a.vi"("error in (no error)"=w300, "Value in"=w302, "Parameter"=w297, "Handle in"=w301) -> ("error out"=w304:errorcluster, "Handle out"=w298:u32)  [unwired: 6 in]
                n91 = call <userlib>:"tm_getparameter_a.vi"("error in (no error)"=w304, "Parameter"=w297, "Handle in"=w298) -> ("error out"=w281:errorcluster, "Value out"=w303:dbl, "Handle out"=w299:u32)  [unwired: 6 in]
                n92 = local read "Internal Line Interval"() -> (w289:dbl)
                n93 = local write "EXP"(w303) -> ()
                n94 = call <userlib>:"tm_setparameter_a.vi"("error in (no error)"=w281, "Value in"=w289, "Parameter"=w296, "Handle in"=w299) -> ("error out"=w282:errorcluster, "Handle out"=w295:u32)  [unwired: 6 in]
                n95 = call <userlib>:"tm_getparameter_a.vi"("error in (no error)"=w282, "Parameter"=w296, "Handle in"=w295) -> ("error out"=w283:errorcluster, "Value out"=w294:dbl, "Handle out"=w293:u32)  [unwired: 6 in]
                n96 = local write "Internal Line Interval"(w294) -> ()
                n97 = local read "Trigger Source"() -> (w288:sgl)
                n98 = call <userlib>:"tm_setparameter_a.vi"("error in (no error)"=w283, "Value in"=w288, "Parameter"=w291, "Handle in"=w293) -> ("error out"=w284:errorcluster, "Handle out"=w292:u32)  [unwired: 6 in]
                n99 = call <userlib>:"tm_getparameter_a.vi"("error in (no error)"=w284, "Parameter"=w291, "Handle in"=w292) -> ("error out"=w285:errorcluster, "Value out"=w290:dbl, "Handle out"=w287:u32)  [unwired: 6 in]
                n100 = local write "Trigger Source"(w290) -> ()
              }
              frame "Idle", Default {
                n101 = call <userlib>:"tm_waitnextframe.vi"("error in (no error)"=w306, "Timeout"=100, "Handle in"=w318) -> ("error out"=w305:errorcluster, "Handle out"=w317:u32)  [unwired: 5 in, 2 out]
                n102 = call <userlib>:"tm_getframe_a.vi"("error in (no error)"=w305, "Buffer Info"=w310, "Handle in"=w317) -> ("error out"=w308:errorcluster, "Data 16"=w312:u16[][], "Handle out"=w309:u32)  [unwired: 4 in, 2 out]
                n103 = Bundle By Name(cluster=w315, "State"=Stack_Track."Idle", "Stack Number"=0, "Image"=w312) -> (w311:cluster{})
                n104 = Enqueue Element(queue=w316, element=w311) -> ()  [unwired: 2 in, 3 out]
              }
            }
            n105 = local read "stop"() -> (w169:bool)
          }
          n106 = while {
            tunnel: w157 -> [w166]
            stop <- "stop" stop-if-true
            n107 = event shown="[0] Timeout" {
              selector: _ -> [_]
              dyn-events: _ -> [_]
              timeout: _ -> [_]
              tunnel: w166 -> [w168]
              event Timeout {
                n108 = event-data() -> ()  [unwired: 1 in, 3 out]
                n109 = Enqueue Element(queue=w168, element=CameraControlTypeDef."Idle") -> ()  [unwired: 2 in, 3 out]
              }
            }
          }
        }
        frame Enabled {
        }
      }
      n110 = while {
        tunnel: w80 -> [w111]
        tunnel: [w109] -> _
        tunnel: [w108] -> w9
        shift-right: [w118] -> _
        shift-left: w79 -> [w116]
        shift-right: [w119] -> _
        shift-left: 0.0 -> [w117]
        shift-right: [w110] -> w10
        shift-left: w79 -> [w114]
        tunnel: w14 -> [w112]
        tunnel: w79 -> [w115]
        shift-right: [w107] -> _
        shift-left: w13 -> [w113]
        shift-right: [w105] -> _
        shift-left: 0 -> [w106]
        tunnel: w15 -> [w104]
        shift-right: [w103] -> _
        shift-left: _ -> [w102]
        tunnel: w12 -> [w101]
        stop <- w120 stop-if-true
        (unwired) 0
        n111 = call <userlib>:"tm_waitnextframe.vi"("error in (no error)"=w111, "Handle in"=w112) -> ("error out"=w94:errorcluster, "Frame Count"=w88:i32, "Frame Index"=w93:i32, "Handle out"=w95:u32)  [unwired: 6 in]
        "Total Frames" <- w88
        n112 = Tick Count (ms)() -> (millisecond timer value=w91:u32)
        n113 = Increment(x=w117) -> (x+1=w89:dbl)
        n114 = Subtract(x=w91, y=w115) -> (x-y=→"Elapsed Time":u32)
        n115 = Add(x=w116, y=u32 1000) -> (x+y=w99:u32)
        n116 = Less Or Equal?(x=w99, y=w91) -> (x <= y?=w90:bool)
        n117 = Add(x=w114, y=u32 50) -> (x+y=w97:u32)
        n118 = Less Or Equal?(x=w97, y=w91) -> (x <= y?=w87:bool)
        n119 = case shown="True" w90 {
          tunnel: w116 -> [w124 w133]
          tunnel: [w124 w130] -> w118
          tunnel: w89 -> [w123 w136]
          tunnel: w91 -> [_ w130]
          tunnel: [w123 0.0] -> w119
          tunnel: w88 -> [_ w125]
          tunnel: w106 -> [w122 w128]
          tunnel: [w122 w125] -> w105
          frame False {
          }
          frame True {
            n120 = Subtract(x=w130, y=w133) -> (x-y=w132:u32)
            n121 = Subtract(x=w125, y=w128) -> (x-y=w126:i32)
            n122 = To Double Precision Float(number=w132) -> (double precision float=w138:dbl)
            n123 = Divide(x=w138, y=1000.0) -> (x/y=w129:dbl)
            n124 = To Double Precision Float(number=w126) -> (double precision float=w127:dbl)
            n125 = Divide(x=w127, y=w129) -> (x/y=→"Camera FPS":dbl)
            n126 = Divide(x=w136, y=w129) -> (x/y=→"Software FPS":dbl)
          }
        }
        n127 = case shown="True" w87 {
          tunnel: w114 -> [w143 _]
          tunnel: w91 -> [_ w156]
          tunnel: [w143 w156] -> w110
          tunnel: w95 -> [w142 w155]
          tunnel: w113 -> [w140 w150]
          tunnel: w94 -> [w141 w154]
          tunnel: [w142 w153] -> w109
          tunnel: [w141 w152] -> w108
          tunnel: w93 -> [_ w151]
          tunnel: [w140 w150] -> w107
          tunnel: w104 -> [_ w149]
          tunnel: w101 -> [_ w145]
          tunnel: [w139 w144] -> w103
          tunnel: w102 -> [w139 _]
          frame False {
          }
          frame True {
            n128 = call <userlib>:"tm_getframe_a.vi"("error in (no error)"=w154, "Frame Index"=w151, "Buffer Info"=w150, "Handle in"=w155) -> ("error out"=w152:errorcluster, "Data 16"=w144:u16[][], "Handle out"=w153:u32)  [unwired: 3 in, 2 out]
            n129 = Bundle By Name(cluster=w145, "State"=Stack_Track."Idle", "Stack Number"=0, "Image"=w144) -> (w146:T3)
            n130 = Enqueue Element(queue=w149, element=w146) -> ()  [unwired: 2 in, 3 out]
          }
        }
        n131 = local read "stop"() -> (w100:bool)
        n132 = Unbundle By Name(w108) -> ("status"=w121:bool)
        n133 = Compound Arithmetic op=OR(w121, w100) -> (w120:bool)
      }
      n134 = while {
        tunnel: w15 -> [w333]
        shift-right: [w329] -> _
        shift-left: _ -> [w327]
        shift-right: [w325] -> _
        shift-left: _ -> [w326]
        shift-right: [w323] -> _
        shift-left: _ -> [w319]
        stop <- w328 stop-if-true
        n135 = Dequeue Element(queue=w333) -> (element=w332:T3, timed out?=w320:bool)  [unwired: 2 in, 2 out]
        n136 = Unbundle By Name(w332) -> ("State"=w331:T1, "Stack Number"=w330:i32, "Image"=w321:u16[][])
        "State" <- w331
        n137 = case shown="False" w320 {
          tunnel: w321 -> [w335 w337]
          tunnel: [w335 w336] -> w322
          tunnel: [w334 w337] -> w323
          tunnel: w319 -> [w334 w336]
          frame False {
          }
          frame True {
          }
        }
        "Image" <- w322
        n138 = case shown="\"Read Disk\"" w331 {
          tunnel: w330 -> [_ _ _ _ _ _]
          tunnel: [w340 w357 _ _ _ _] -> w329
          tunnel: w327 -> [_ w358 w362 _ _ _]
          tunnel: [FALSE _ _ _ TRUE _] -> w328
          tunnel: w322 -> [w338 w359 _ _ _ _]
          tunnel: w326 -> [_ w356 w360 w369 w394 w396]
          tunnel: [w341 w355 w361 w366 w394 w396] -> w325
          tunnel: "Path" -> [w344 _ _ w371 _ _]
          frame "Start Sequence" {
            # "Public tiff library"
            # "Get path and open file"
            n139 = Equal?(x=w344, y=path "") -> (x = y?=w346:bool)
            n140 = case shown="True" w346 {
              tunnel: w344 -> [w348 _]
              tunnel: [w348 w351] -> w343
              frame False {
              }
              frame True {
                n141 = call "File Dialog"("pattern (all files)"=".tiff", "pattern label"="Tiff Image") -> ("selected path"=w351:path)  [unwired: 10 in, 3 out]
              }
            }
            n142 = case shown="False" "AutoIncrement" {
              tunnel: w343 -> [w352 w354]
              tunnel: [w352 w353] -> w339
              frame False {
              }
              frame True {
                n143 = call "4Digit File Incrementer.vi"("path"=w354) -> ("appended path"=w353:path)  [unwired: 10 in]
              }
            }
            n144 = call-poly "CTIFFNewFileAndStyle.vi"("image"=w338, "output_file"=w339) -> ("error"=w341:errorcluster, "CTIFF"=w340:i64)  [unwired: 8 in]
            n145 = local write "Path"(w339) -> ()
          }
          frame "Collecting" {
            (unwired) "Saving" ("Boolean Text.Text")
            (unwired) T8."Disabled and Grayed Out" ("Disabled")
            # "Add Image to write scan line"
            n146 = call-poly "CTIFFAddNewPage.vi"("error"=w356, "image"=w359, "CTIFF"=w358) -> ("error"=w355:errorcluster, "CTIFF"=w357:i64)  [unwired: 7 in]
          }
          frame "End" {
            (unwired) "OK" ("Boolean Text.Text")
            (unwired) T8."Enabled" ("Disabled")
            (unwired) FALSE
            # "Close image file, reset capturing button"
            n147 = call "CTIFFWriteAndClose.vi"("error"=w360, "CTIFF"=w362) -> ("error"=w361:errorcluster)  [unwired: 9 in]
          }
          frame "Read Disk" {
            n148 = call <userlib>:"tm_opendcimgfile.vi"() -> ("Total Frames"=w372:i32, "File Handle"=w373:u32)  [unwired: 9 in, 1 out]
            n149 = for {
              N: w372 -> [_]
              tunnel: w371 -> [w381]
              shift-right: [w379] -> w367
              shift-left: i64 0 ("CTIFF") -> [w380]
              tunnel: [w378] -> w368
              tunnel: w369 -> [w377]
              shift-right: [w383] -> w363
              shift-left: w373 -> [w384]
              i -> [w375]
              n150 = Equal To 0?(x=w375) -> (x = 0?=w382:bool)
              n151 = call <userlib>:"tm_getdcimgframe.vi"("error in (no error)"=w377, "Frame Index"=w375, "File Handle in"=w384) -> ("error out"=w376:errorcluster, "Data"=w374:u16[][], "File Handle out"=w383:u32)  [unwired: 5 in, 1 out]
              n152 = local write "Image"(w374) -> ()
              n153 = case shown="True" w382 {
                tunnel: w381 -> [_ w393]
                tunnel: w374 -> [w385 w392]
                tunnel: w380 -> [w389 _]
                tunnel: [w388 w391] -> w379
                tunnel: [w387 w390] -> w378
                tunnel: w376 -> [w386 _]
                frame False {
                  n154 = call-poly "CTIFFAddNewPage.vi"("error"=w386, "image"=w385, "CTIFF"=w389) -> ("error"=w387:errorcluster, "CTIFF"=w388:i64)  [unwired: 7 in]
                }
                frame True {
                  n155 = call-poly "CTIFFNewFileAndStyle.vi"("image"=w392, "output_file"=w393) -> ("error"=w390:errorcluster, "CTIFF"=w391:i64)  [unwired: 8 in]
                }
              }
              "Frame Index" <- w375
            }
            n156 = call "CTIFFWriteAndClose.vi"("error"=w368, "CTIFF"=w367) -> ("error"=w365:errorcluster)  [unwired: 9 in]
            n157 = call <userlib>:"tm_closedcimgfile.vi"("error in (no error)"=w365, "File Handle"=w363) -> ("error out"=w364:errorcluster)  [unwired: 9 in]
            n158 = Delete(error in=w364) -> (error out=w366:errorcluster)  [unwired: 4 in, 2 out]
          }
          frame "STOP" {
          }
          frame "Idle" {
          }
        }
      }
      n159 = call <userlib>:"tm_stopcapture.vi"("error in (no error)"=w9, "Handle in"=w10) -> ("error out"=w55:errorcluster, "Handle out"=w56:u32)  [unwired: 8 in]
      n160 = call <userlib>:"tm_unpreparecapture.vi"("error in (no error)"=w55, "Handle in"=w56) -> ("error out"=w54:errorcluster, "Handle out"=w57:u32)  [unwired: 8 in]
      n161 = call <userlib>:"tm_closecamera.vi"("error in (no error)"=w54, "Handle in"=w57) -> ("error out"=w84:errorcluster)  [unwired: 9 in]
      n162 = call <userlib>:"tm_deinitialize.vi"("error in (no error)"=w84) -> ("error out"=w83:errorcluster)  [unwired: 10 in]
    }
  }
  "error out" <- w3
